vi "main init.vi"(8 "error in (no error)":errorcluster) -> (0 "error out":errorcluster, 3 "position out":cluster{"x":dbl, "y":dbl, "degree":dbl})   [LabVIEW 2019]
uses:
  servo state.ctl
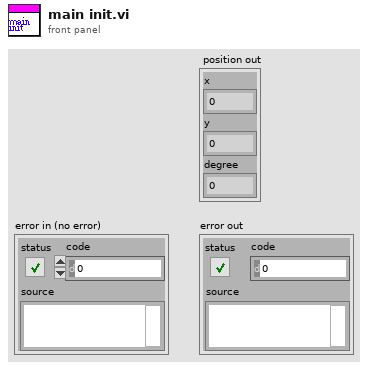
[diagram p1: front panel]
types:
  T1 = typedef "servo state.ctl" = enum16{"catch", "cam-1", "put", "side", "center", "side-2", "put-2"}
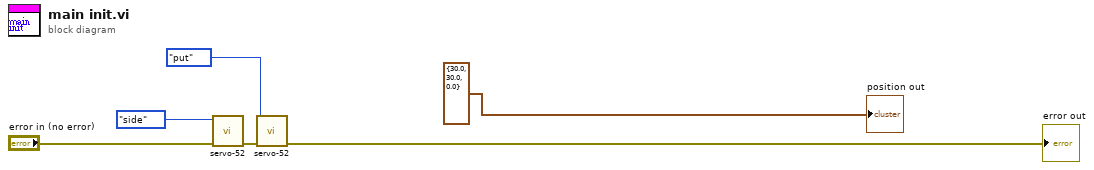
[diagram p0: block diagram]
diagram:
  n1 = call "servo-52.vi"("error in (no error)"="error in (no error)", "Enum"=servo_state."side") -> ("error out"=w4:errorcluster)  [unwired: 9 in]
  n2 = call "servo-52.vi"("error in (no error)"=w4, "Enum"=servo_state."put") -> ("error out"=→"error out":errorcluster)  [unwired: 9 in]
  "position out" <- cluster{"x":dbl, "y":dbl, "degree":dbl} {"x"=30.0, "y"=30.0, "degree"=0.0} ("position out")
